vi "Is Pin or Relay Name in Map.vi"(8 "error in":errorcluster, 10 "pin or relay name":string, 11 "connection map in":refnum<class "Connection Map.lvclass">) -> (0 "error out":errorcluster, 2 "pin or relay name in map":bool, 3 "connection map out":refnum<class "Connection Map.lvclass">)   [LabVIEW 2020, in "Measurement Plugin Session Management V1.lvlib" / "Connection Map.lvclass"]
uses:
  Connection Map.lvclass
  Connection Map.lvclass/Connection Map.ctl
  fcefb7b9-c03e-4452-965d-690b73631330.vi
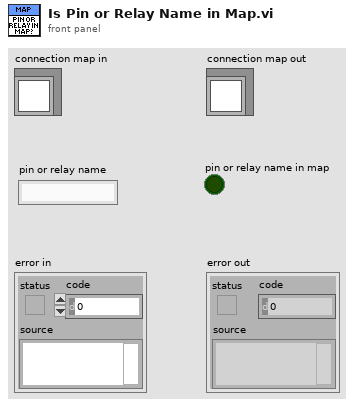
[diagram p1: front panel]
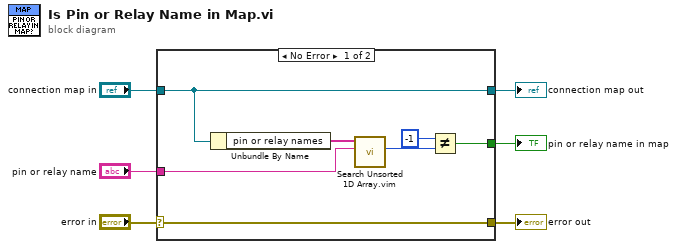
[diagram p0: block diagram]
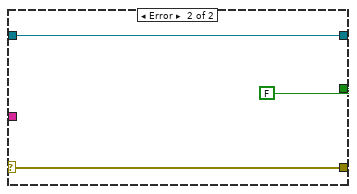
[diagram p2: hidden frame]
diagram:
  n1 = case shown="No Error" "error in" {
    selector: "error in" -> [w13 w16]
    tunnel: [w13 w16] -> w5
    tunnel: [w12 w15] -> w3
    tunnel: "connection map in" -> [w12 w15]
    tunnel: "pin or relay name" -> [w10 _]
    tunnel: [w7 FALSE ("key not found?")] -> w1
    frame No Error {
      n2 = Unbundle By Name(w12) -> ("pin or relay names"=w11:string[])
      n3 = call "Search Unsorted 1D Array.vim"("element"=w10, "unsorted 1D array"=w11) -> ("index of element"=w9:i32)  [unwired: 9 in]
      n4 = Not Equal?(x=-1, y=w9) -> (x != y?=w7:bool)
    }
    frame Error {
    }
  }
  "error out" <- w5
  "connection map out" <- w3
  "pin or relay name in map" <- w1
